vi "Configure Memory.vi"(0 "VISA resource name":refnum<visa-resource-name>, 5 "File Type (2: Event)":u16(ring)=2 items=["Display", "Display + Event", "Event"], 11 "error in (no error)":errorcluster) -> (4 "VISA resource name out":refnum<visa-resource-name>, 15 "error out":errorcluster)   [LabVIEW 2020, in "Yokogawa GX Series.lvlib"]
doc: "Sets the type of data to record.\n\nCommand: SMemory"
uses:
  <instrlib>/Yokogawa GX Series/Yokogawa GX Series.lvlib
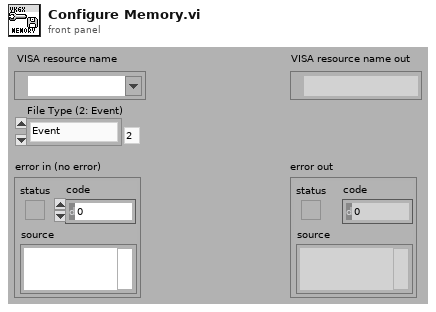
[diagram p1: front panel]
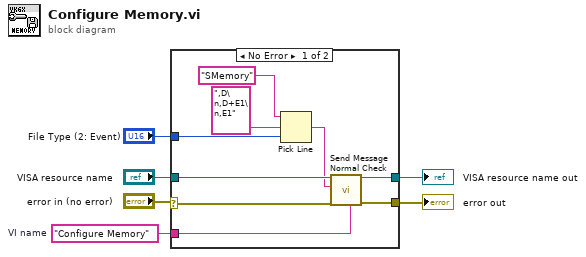
[diagram p0: block diagram]
diagram:
  w5 = "Configure Memory"  # VI name
  n1 = case shown="No Error" "error in (no error)" {
    selector: "error in (no error)" -> [w8 w16]
    tunnel: "VISA resource name" -> [w15 w17]
    tunnel: w5 -> [w7 _]
    tunnel: [w14 w17] -> w4
    tunnel: [w13 w16] -> w3
    tunnel: "File Type (2: Event)" -> [w12 _]
    frame No Error {
      n2 = Pick Line(string ("")="SMemory", multi-line string=",D\n,D+E1\n,E1", line index=w12) -> (output string=w10:string)
      n3 = call <instrlib>:"Send Message Normal Check.vi"("Source (\"\")"=w7, "error in (no error)"=w8, "Send Message (\"\")"=w10, "VISA resource name"=w15) -> ("error out"=w13:errorcluster, "VISA resource name out"=w14:refnum<visa-resource-name>)  [unwired: 2 in, 4 out]
    }
    frame Error {
    }
  }
  "error out" <- w3
  "VISA resource name out" <- w4
